vi "Merge AO Settings from Generator.vi"(8 "error in (no error)":errorcluster, 10 "configuration.AO Channels":T1, 11 "Instrument.DAQ in":refnum<class "Instrument.DAQ.lvclass">) -> (0 "error out":errorcluster, 3 "Instrument.DAQ out":refnum<class "Instrument.DAQ.lvclass">)   [LabVIEW 2019, in "Instrument.Lockin.lvlib" / "Instrument.DAQ.lvclass"]
uses:
  Instrument.DAQ.lvclass
  Generator/typedefs/AO.Channel--Cluster--Array.ctl
  Generator/typedefs/AO.Channel--Cluster.ctl
  Generator/typedefs/AO.Channel.Function--Enum.ctl
  Instrument.DAQ.lvclass/Instrument.DAQ.ctl
  Typedefs/AO.Channel--Cluster.ctl
  Typedefs/AO.Channel.Function--Enum.ctl
  Generator/Generator.lvclass
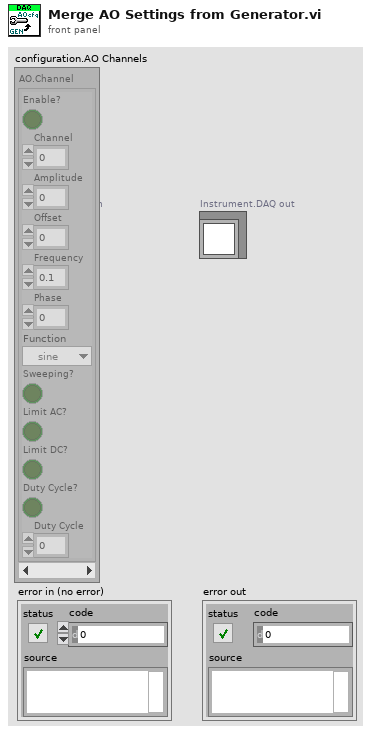
[diagram p1: front panel]
types:
  T1 = typedef "Generator.lvclass/AO.Channel--Cluster--Array.ctl" = T2[]
  T2 = typedef "Generator.lvclass/AO.Channel--Cluster.ctl" = cluster{"Enable?":bool, "Channel":i32, "Amplitude":dbl, "Offset":dbl, "Frequency":dbl, "Phase":dbl, "Function":T3, "Sweeping?":bool, "Limit AC?":bool, "Limit DC?":bool, "Duty Cycle?":bool, "Duty Cycle":dbl}
  T3 = typedef "Generator.lvclass/AO.Channel.Function--Enum.ctl" = enum16{"sine", "square", "triangle", "saw"}
  T4 = typedef "Instrument.Lockin.lvlib/Instrument.DAQ.lvclass/AO.Channel--Cluster--Array.ctl" = T5[]
  T5 = typedef "Instrument.Lockin.lvlib/Instrument.DAQ.lvclass/AO.Channel--Cluster.ctl" = cluster{"Enable?":bool, "Channel":i32, "Amplitude":dbl, "Offset":dbl, "Frequency":dbl, "Phase":dbl, "Function":T6, "Sweeping?":bool, "Limit AC":bool, "Limit DC?":bool, "Duty Cycle":bool}
  T6 = typedef "Instrument.Lockin.lvlib/Instrument.DAQ.lvclass/AO.Channel.Function--Enum.ctl" = enum16{"sine", "square", "triangle", "saw"}
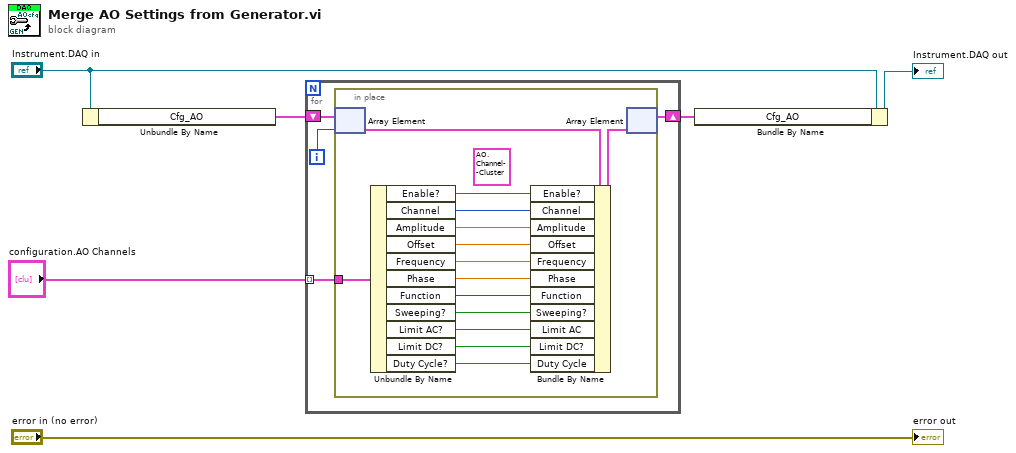
[diagram p0: block diagram]
diagram:
  n1 = Unbundle By Name("Instrument.DAQ in") -> ("Cfg_AO"=w2:T4)
  n2 = for {
    tunnel: "configuration.AO Channels" -> [w10] mode=indexing
    shift-right: [w7] -> w1
    shift-left: w2 -> [w9]
    i -> [w8]
    n3 = in-place {
      in-place-border: w10 -> [w13]
      (unwired) T5 {"Enable?"=TRUE, "Channel"=0, "Amplitude"=0.0, "Offset"=0.0, "Frequency"=10.0, "Phase"=0.0, "Function"=enum."sine", "Sweeping?"=TRUE, "Limit AC"=TRUE, "Limit DC?"=TRUE, "Duty Cycle"=TRUE} ("input cluster")
      n4 = in-place-array #1(w9, w8) -> (w11:T5)
      n5 = Unbundle By Name(w13) -> ("Enable?"=w24:bool, "Channel"=w15:i32, "Amplitude"=w16:dbl, "Offset"=w17:dbl, "Frequency"=w18:dbl, "Phase"=w19:dbl, "Function"=w14:T3, "Sweeping?"=w20:bool, "Limit AC?"=w21:bool, "Limit DC?"=w22:bool, "Duty Cycle?"=w23:bool)
      n6 = Bundle By Name(cluster=w11, "Enable?"=w24, "Channel"=w15, "Amplitude"=w16, "Offset"=w17, "Frequency"=w18, "Phase"=w19, "Function"=w14, "Sweeping?"=w20, "Limit AC"=w21, "Limit DC?"=w22, "Duty Cycle"=w23) -> (w12:T5)
      n7 = in-place-array #1(w12) -> (w7:T4)  [unwired: 1 out]
    }
  }
  n8 = Bundle By Name(cluster="Instrument.DAQ in", "Cfg_AO"=w1) -> (→"Instrument.DAQ out":refnum<class "Instrument.DAQ.lvclass">)
  "error out" <- "error in (no error)"
